vi "_PC_Pub_ExpCondi exportToArray.vi"(1 "ExpCondi":T1=[{"Label"="Laser", "Value"=variant}, {"Label"="Pressure", "Value"=variant}, {"Label"="TMP", "Value"=variant}, {"Label"="Script", "Value"=variant}, {"Label"="Signal Remarks", "Value"=variant}, {"Label"="ExtAO", "Value"=variant}, {"Label"="ExtDO", "Value"=variant}, {"Label"="ExtDI", "Value"=variant}, {"Label"="D999", "Value"=variant}]) -> (0 "appended array":string[][](array[string]))   [LabVIEW 2018]
uses:
  RT/PublicSubVI/Ctl/_ctl_RT_ExpCondi.ctl
  RT/PublicSubVI/Ctl/_ctl_RT_ExtAO.ctl
  RT/PublicSubVI/Ctl/_ctl_RT_extDO.ctl
  RT/PublicSubVI/Ctl/_ctl_RT_extDI.ctl
  RT/PublicSubVI/Ctl/_ctl_RT_D999_Format.ctl
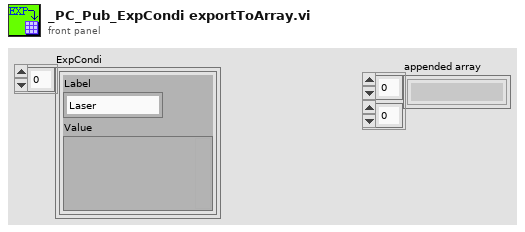
[diagram p1: front panel]
types:
  T1 = typedef "_ctl_RT_ExpCondi.ctl" = cluster{"Label":string, "Value":variant}[]
  T2 = cluster{"Label":string, "dt":dbl, "ScanRate":dbl, "mz0":dbl, "Length":u32, "RefVolt":dbl}[]
  T3 = typedef "_ctl_RT_ExtAO.ctl" = cluster{"Label":string, "y":dbl}[]
  T4 = typedef "_ctl_RT_extDO.ctl" = cluster{"Label":string, "Boolean":bool}[]
  T5 = typedef "_ctl_RT_extDI.ctl" = cluster{"Label":string}[]
  T6 = typedef "_ctl_RT_D999_Format.ctl" = cluster{"Port":string, "Label":string, "Value":dbl}[]
  T7 = cluster{"param":cluster{"label":string, "data":string}[], "code":string}
  T8 = cluster{"DiodeTemp":dbl, "SHGTemp":dbl, "THGTemp":dbl, "HeadTemp":dbl, "DiodeHour":dbl, "PulseCount":dbl, "PulseEnergy":dbl, "Actual Freq":dbl, "Actual Current%":dbl}
  T9 = typedef "Type Descriptor Enumeration__ogtk.ctl" = enum8{"<Null>", "I8", "I16", "I32", "I64", "U8", "U16", "U32", "U64", "SGL", "DBL", "EXT", "CSG", "CDB", "CXT", "0x0F", "0x10", "0x11", "0x12", "0x13", "0x14", "Enum U8", "Enum U16", "Enum U32", "Enum U64", "SGL PQ", "DBL PQ", "EXT PQ", "CSG PQ", "CDB PQ", "CXT PQ", "0x1F", "0x20", "Boolean", "0x22", "0x23", "0x24", "0x25", "0x26", "0x27", "0x28", "0x29", "0x2A", "0x2B", "0x2C", "0x2D", "0x2E", "0x2F", "String", "0x31", "Path", "Pict", "0x34", "0x35", "0x36", "DAQ", "0x38", "0x39", "0x3A", "0x3B", "0x3C", "0x3D", "0x3E", "0x3F", "Array", "0x41", "0x42", "0x43", "0x44", "0x45", "0x46", "0x47", "0x48", "0x49", "0x4A", "0x4B", "0x4C", "0x4D", "0x4E", "0x4F", "Cluster", "0x51", "0x52", "Variant", "Waveform", "0x55", "0x56", "0x57", "0x58", "0x59", "0x5A", "0x5B", "0x5C", "0x5D", "0x5E", "0x5F", "0x60", "0x61", "0x62", "0x63", "0x64", "0x65", "0x66", "0x67", "0x68", "0x69", "0x6A", "0x6B", "0x6C", "0x6D", "0x6E", "0x6F", "Refnum"}
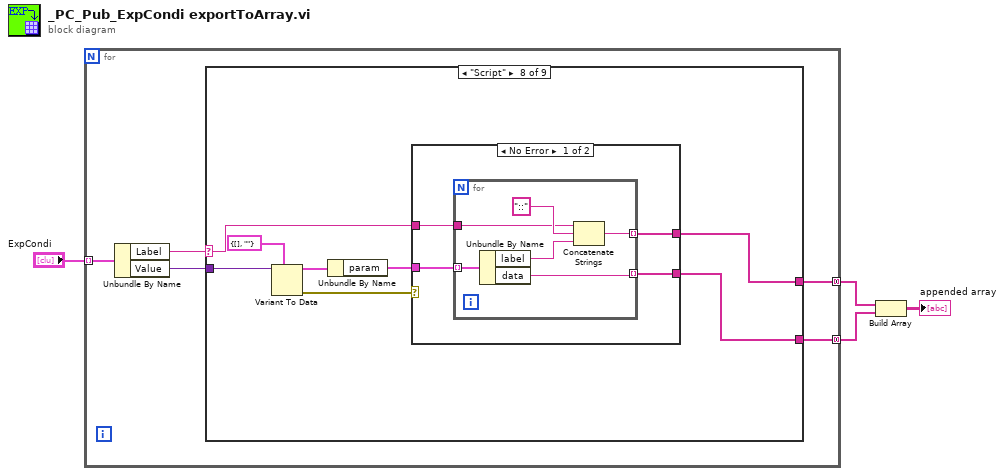
[diagram p0: block diagram]
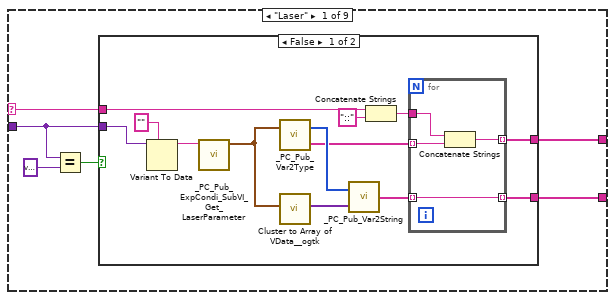
[diagram p2: hidden frame]
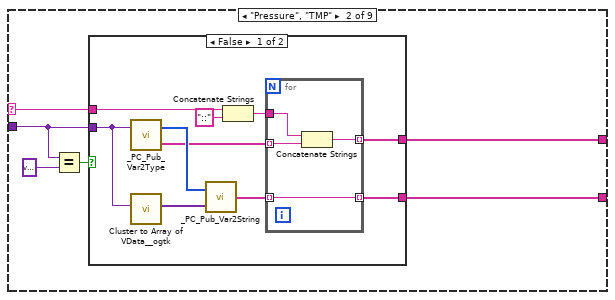
[diagram p4: hidden frame]
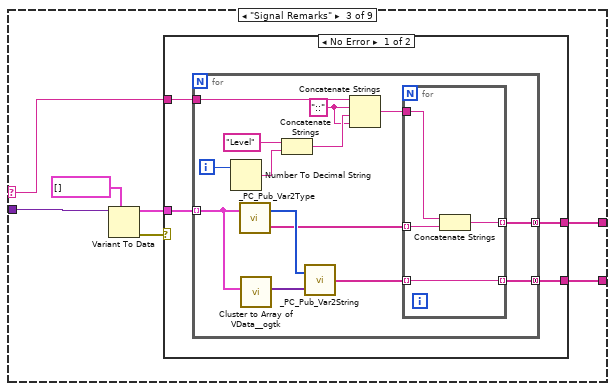
[diagram p6: hidden frame]
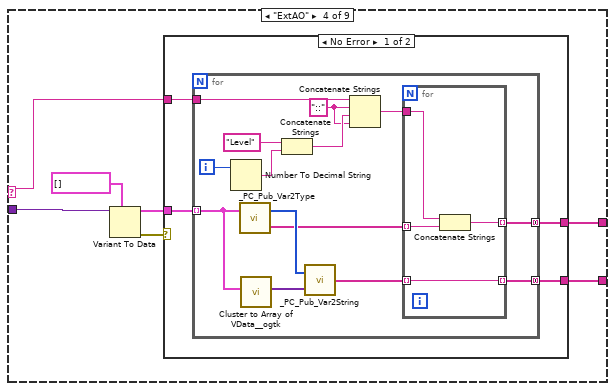
[diagram p8: hidden frame]
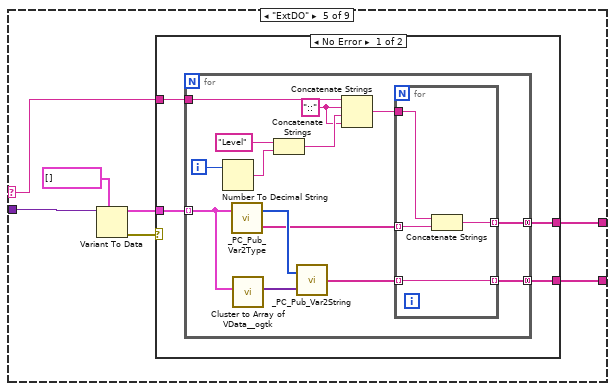
[diagram p10: hidden frame]
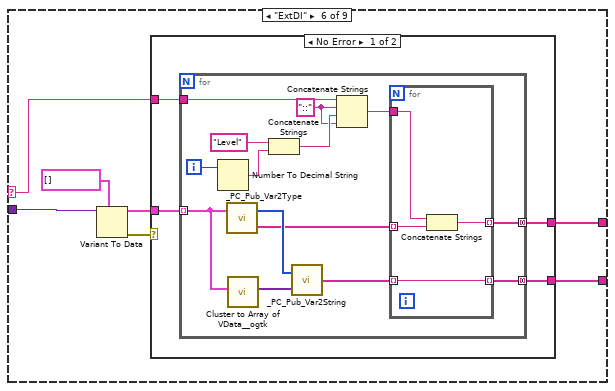
[diagram p12: hidden frame]
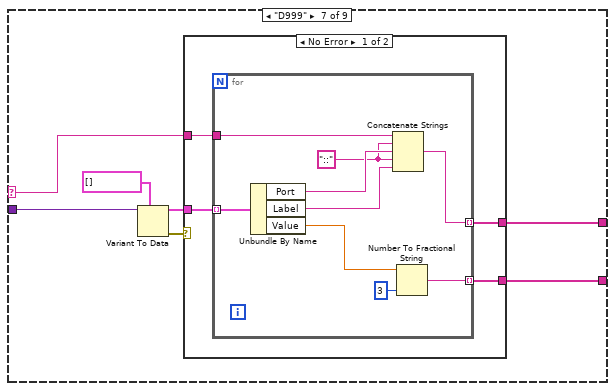
[diagram p14: hidden frame]
diagram:
  n1 = for {
    tunnel: [w9] -> w4 mode=concatenating
    tunnel: [w8] -> w3 mode=concatenating
    tunnel: "ExpCondi" -> [w7] mode=indexing
    n2 = Unbundle By Name(w7) -> ("Label"=w5:string, "Value"=w6:variant)
    n3 = case shown="\"Script\"" w5 {
      selector: w5 -> [w13 w36 w53 w82 w111 w140 w169 w191 _]
      tunnel: w6 -> [w12 w35 w54 w88 w117 w146 w175 w196 _]
      tunnel: [w11 w37 w56 w85 w114 w143 w171 w190 _] -> w9
      tunnel: [w10 w38 w57 w86 w115 w144 w170 w189 _] -> w8
      frame "Laser" {
        n4 = Equal?(x=w12, y=variant) -> (x = y?=w14:bool)
        n5 = case shown="False" w14 {
          tunnel: [w28 _] -> w10
          tunnel: [w27 _] -> w11
          tunnel: w13 -> [w26 _]
          tunnel: w12 -> [w22 _]
          frame False {
            n6 = Variant To Data(type="", Variant=w22) -> (data=w20:string)  [unwired: 1 in, 1 out]
            n7 = call "_PC_Pub_ExpCondi_SubVI_Get_LaserParameter.vi"("result string"=w20) -> ("output cluster"=w17:T8)  [unwired: 9 in, 1 out]
            n8 = call "_PC_Pub_Var2Type.vi"("Input Variable"=w17) -> ("Output Name"=w18:string[], "Output Type"=w19:T9[])  [unwired: 1 in]
            n9 = call <userlib>:"Cluster to Array of VData__ogtk.vi"("Cluster"=w17) -> ("Array of VData"=w16:variant[])  [unwired: 9 in, 1 out]
            n10 = call "_PC_Pub_Var2String.vi"("Array of VData"=w16, "Output Type"=w19) -> ("String Array"=w25:string[])
            n11 = Concatenate Strings(w26, "::" ("string")) -> (w23:string)
            n12 = for {
              tunnel: w25 -> [w30] mode=indexing
              tunnel: w18 -> [w31] mode=indexing
              tunnel: w23 -> [w32]
              tunnel: [w30] -> w28 mode=indexing
              tunnel: [w29] -> w27 mode=indexing
              n13 = Concatenate Strings(w32, w31) -> (w29:string)
            }
          }
          frame True {
          }
        }
      }
      frame "Pressure", "TMP" {
        n14 = Equal?(x=w35, y=variant) -> (x = y?=w33:bool)
        n15 = case shown="False" w33 {
          tunnel: [w48 _] -> w38
          tunnel: [w47 _] -> w37
          tunnel: w36 -> [w44 _]
          tunnel: w35 -> [w39 _]
          frame False {
            n16 = call "_PC_Pub_Var2Type.vi"("Input Variable"=w39) -> ("Output Name"=w45:string[], "Output Type"=w46:T9[])  [unwired: 1 in]
            n17 = call <userlib>:"Cluster to Array of VData__ogtk.vi"("Cluster"=w39) -> ("Array of VData"=w43:variant[])  [unwired: 9 in, 1 out]
            n18 = call "_PC_Pub_Var2String.vi"("Array of VData"=w43, "Output Type"=w46) -> ("String Array"=w42:string[])
            n19 = Concatenate Strings(w44, "::" ("string")) -> (w40:string)
            n20 = for {
              tunnel: w42 -> [w50] mode=indexing
              tunnel: w45 -> [w51] mode=indexing
              tunnel: w40 -> [w52]
              tunnel: [w50] -> w48 mode=indexing
              tunnel: [w49] -> w47 mode=indexing
              n21 = Concatenate Strings(w52, w51) -> (w49:string)
            }
          }
          frame True {
          }
        }
      }
      frame "Signal Remarks" {
        n22 = Variant To Data(type=T2 [] ("Signal Remarks"), Variant=w54) -> (data=w58:T2, error out=w55:errorcluster)  [unwired: 1 in]
        n23 = case shown="No Error" w55 {
          tunnel: w58 -> [w63 _]
          tunnel: [w62 _] -> w57
          tunnel: [w61 _] -> w56
          tunnel: w53 -> [w60 _]
          frame No Error {
            n24 = for {
              tunnel: w63 -> [w77] mode=indexing
              tunnel: [w71] -> w61 mode=concatenating
              tunnel: [w70] -> w62 mode=concatenating
              tunnel: w60 -> [w64]
              i -> [w67]
              w65 = "::" ("string")
              n25 = Number To Decimal String(number=w67) -> (decimal integer string=w69:string)  [unwired: 1 in]
              n26 = call "_PC_Pub_Var2Type.vi"("Input Variable"=w77) -> ("Output Name"=w74:string[], "Output Type"=w75:T9[])  [unwired: 1 in]
              n27 = call <userlib>:"Cluster to Array of VData__ogtk.vi"("Cluster"=w77) -> ("Array of VData"=w76:variant[])  [unwired: 9 in, 1 out]
              n28 = Concatenate Strings("Level", w69) -> (w66:string)
              n29 = call "_PC_Pub_Var2String.vi"("Array of VData"=w76, "Output Type"=w75) -> ("String Array"=w73:string[])
              n30 = Concatenate Strings(w64, w65, w66, w65) -> (w72:string)
              n31 = for {
                tunnel: w73 -> [w78] mode=indexing
                tunnel: w74 -> [w80] mode=indexing
                tunnel: w72 -> [w81]
                tunnel: [w79] -> w71 mode=indexing
                tunnel: [w78] -> w70 mode=indexing
                n32 = Concatenate Strings(w81, w80) -> (w79:string)
              }
            }
          }
          frame Error {
          }
        }
      }
      frame "ExtAO" {
        n33 = Variant To Data(type=T3 [] ("ExtAO"), Variant=w88) -> (data=w87:T3, error out=w84:errorcluster)  [unwired: 1 in]
        n34 = case shown="No Error" w84 {
          tunnel: w87 -> [w92 _]
          tunnel: [w91 _] -> w86
          tunnel: [w90 _] -> w85
          tunnel: w82 -> [w89 _]
          frame No Error {
            n35 = for {
              tunnel: w92 -> [w106] mode=indexing
              tunnel: [w100] -> w90 mode=concatenating
              tunnel: [w99] -> w91 mode=concatenating
              tunnel: w89 -> [w93]
              i -> [w96]
              w94 = "::" ("string")
              n36 = Number To Decimal String(number=w96) -> (decimal integer string=w98:string)  [unwired: 1 in]
              n37 = call "_PC_Pub_Var2Type.vi"("Input Variable"=w106) -> ("Output Name"=w103:string[], "Output Type"=w104:T9[])  [unwired: 1 in]
              n38 = call <userlib>:"Cluster to Array of VData__ogtk.vi"("Cluster"=w106) -> ("Array of VData"=w105:variant[])  [unwired: 9 in, 1 out]
              n39 = Concatenate Strings("Level", w98) -> (w95:string)
              n40 = call "_PC_Pub_Var2String.vi"("Array of VData"=w105, "Output Type"=w104) -> ("String Array"=w102:string[])
              n41 = Concatenate Strings(w93, w94, w95, w94) -> (w101:string)
              n42 = for {
                tunnel: w102 -> [w107] mode=indexing
                tunnel: w103 -> [w109] mode=indexing
                tunnel: w101 -> [w110]
                tunnel: [w108] -> w100 mode=indexing
                tunnel: [w107] -> w99 mode=indexing
                n43 = Concatenate Strings(w110, w109) -> (w108:string)
              }
            }
          }
          frame Error {
          }
        }
      }
      frame "ExtDO" {
        n44 = Variant To Data(type=T4 [] ("ExtDO"), Variant=w117) -> (data=w116:T4, error out=w113:errorcluster)  [unwired: 1 in]
        n45 = case shown="No Error" w113 {
          tunnel: w116 -> [w121 _]
          tunnel: [w120 _] -> w115
          tunnel: [w119 _] -> w114
          tunnel: w111 -> [w118 _]
          frame No Error {
            n46 = for {
              tunnel: w121 -> [w135] mode=indexing
              tunnel: [w129] -> w119 mode=concatenating
              tunnel: [w128] -> w120 mode=concatenating
              tunnel: w118 -> [w122]
              i -> [w125]
              w123 = "::" ("string")
              n47 = Number To Decimal String(number=w125) -> (decimal integer string=w127:string)  [unwired: 1 in]
              n48 = call "_PC_Pub_Var2Type.vi"("Input Variable"=w135) -> ("Output Name"=w132:string[], "Output Type"=w133:T9[])  [unwired: 1 in]
              n49 = call <userlib>:"Cluster to Array of VData__ogtk.vi"("Cluster"=w135) -> ("Array of VData"=w134:variant[])  [unwired: 9 in, 1 out]
              n50 = Concatenate Strings("Level", w127) -> (w124:string)
              n51 = call "_PC_Pub_Var2String.vi"("Array of VData"=w134, "Output Type"=w133) -> ("String Array"=w131:string[])
              n52 = Concatenate Strings(w122, w123, w124, w123) -> (w130:string)
              n53 = for {
                tunnel: w131 -> [w136] mode=indexing
                tunnel: w132 -> [w138] mode=indexing
                tunnel: w130 -> [w139]
                tunnel: [w137] -> w129 mode=indexing
                tunnel: [w136] -> w128 mode=indexing
                n54 = Concatenate Strings(w139, w138) -> (w137:string)
              }
            }
          }
          frame Error {
          }
        }
      }
      frame "ExtDI" {
        n55 = Variant To Data(type=T5 [] ("ExtDI"), Variant=w146) -> (data=w145:T5, error out=w142:errorcluster)  [unwired: 1 in]
        n56 = case shown="No Error" w142 {
          tunnel: w145 -> [w150 _]
          tunnel: [w149 _] -> w144
          tunnel: [w148 _] -> w143
          tunnel: w140 -> [w147 _]
          frame No Error {
            n57 = for {
              tunnel: w150 -> [w164] mode=indexing
              tunnel: [w158] -> w148 mode=concatenating
              tunnel: [w157] -> w149 mode=concatenating
              tunnel: w147 -> [w151]
              i -> [w154]
              w152 = "::" ("string")
              n58 = Number To Decimal String(number=w154) -> (decimal integer string=w156:string)  [unwired: 1 in]
              n59 = call "_PC_Pub_Var2Type.vi"("Input Variable"=w164) -> ("Output Name"=w161:string[], "Output Type"=w162:T9[])  [unwired: 1 in]
              n60 = call <userlib>:"Cluster to Array of VData__ogtk.vi"("Cluster"=w164) -> ("Array of VData"=w163:variant[])  [unwired: 9 in, 1 out]
              n61 = Concatenate Strings("Level", w156) -> (w153:string)
              n62 = call "_PC_Pub_Var2String.vi"("Array of VData"=w163, "Output Type"=w162) -> ("String Array"=w160:string[])
              n63 = Concatenate Strings(w151, w152, w153, w152) -> (w159:string)
              n64 = for {
                tunnel: w160 -> [w165] mode=indexing
                tunnel: w161 -> [w167] mode=indexing
                tunnel: w159 -> [w168]
                tunnel: [w166] -> w158 mode=indexing
                tunnel: [w165] -> w157 mode=indexing
                n65 = Concatenate Strings(w168, w167) -> (w166:string)
              }
            }
          }
          frame Error {
          }
        }
      }
      frame "D999" {
        n66 = Variant To Data(type=T6 [] ("EC Format"), Variant=w175) -> (data=w173:T6, error out=w172:errorcluster)  [unwired: 1 in]
        n67 = case shown="No Error" w172 {
          tunnel: w173 -> [w179 _]
          tunnel: [w178 _] -> w170
          tunnel: [w177 _] -> w171
          tunnel: w169 -> [w176 _]
          frame No Error {
            n68 = for {
              tunnel: w179 -> [w188] mode=indexing
              tunnel: [w183] -> w177 mode=indexing
              tunnel: [w181] -> w178 mode=indexing
              tunnel: w176 -> [w185]
              w184 = "::" ("string")
              n69 = Unbundle By Name(w188) -> ("Port"=w187:string, "Label"=w186:string, "Value"=w182:dbl)
              n70 = Concatenate Strings(w185, w184, w187, w184, w186) -> (w183:string)
              n71 = Number To Fractional String(number=w182, precision (6)=i16 3) -> (F-format string=w181:string)  [unwired: 2 in]
            }
          }
          frame Error {
          }
        }
      }
      frame "Script" {
        n72 = Variant To Data(type=T7 {"param"=[], "code"=""} ("Script"), Variant=w196) -> (data=w193:T7, error out=w194:errorcluster)  [unwired: 1 in]
        n73 = Unbundle By Name(w193) -> ("param"=w192:cluster{"label":string, "data":string}[])
        n74 = case shown="No Error" w194 {
          tunnel: w192 -> [w200 _]
          tunnel: w191 -> [w199 _]
          tunnel: [w198 _] -> w189
          tunnel: [w197 _] -> w190
          frame No Error {
            n75 = for {
              tunnel: w200 -> [w204] mode=indexing
              tunnel: w199 -> [w205]
              tunnel: [w202] -> w197 mode=indexing
              tunnel: [w201] -> w198 mode=indexing
              n76 = Unbundle By Name(w204) -> ("label"=w203:string, "data"=w201:string)
              n77 = Concatenate Strings(w205, "::" ("string"), w203) -> (w202:string)
            }
          }
          frame Error {
          }
        }
      }
      frame "None", Default {
      }
    }
  }
  n78 = Build Array(w4, w3) -> (→"appended array":string[][])
